vi "Query Event Log Last Entry.vi"(8 "error in (no error)":errorcluster, 11 "VISA resource name":refnum<visa-resource-name>) -> (0 "error out":errorcluster, 1 "Timestamp":string, 2 "Severity":i32, 3 "VISA resource name out":refnum<visa-resource-name>, 4 "Message":string)   [LabVIEW 2020, in "Rohde&Schwarz CMXP Base.lvlib"]
doc: "Queries the last event log.\n\nAttribute:\nRSCMXPBASE_ATTR_EVENT_LOG_LAST_ENTRIES\n\nRemote-control command:\nSENSe:ELOG:LAST?"
uses:
  <instrlib>/Rohde&Schwarz CMXP Base/Rohde&Schwarz CMXP Base.lvlib
  <instrlib>/Rohde&Schwarz CMXP Base/Private/rsidr_core.llb/rsidr_core.lvlib
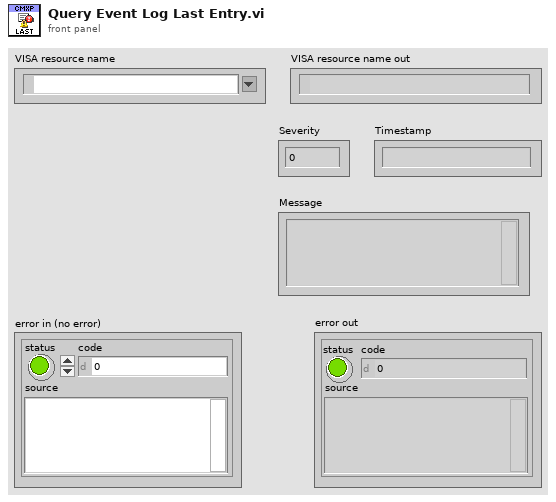
[diagram p1: front panel]
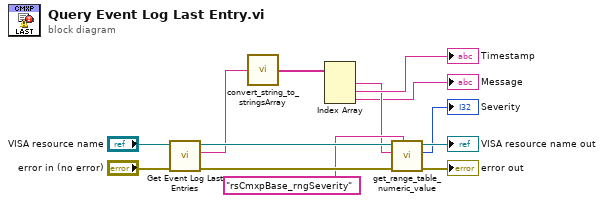
[diagram p0: block diagram]
diagram:
  n1 = call "Get Event Log Last Entries"("error in (no error)"="error in (no error)", "instrument handle"="VISA resource name") -> ("error out"=w8:errorcluster, "Event Log Last Entries"=w3:string, "instrument handle out"=w7:refnum<visa-resource-name>)  [unwired: 7 in]
  n2 = call <instrlib>:"convert_string_to_stringsArray.vi"("String in"=w3) -> ("string array out"=w5:string[])  [unwired: 3 in, 1 out]
  n3 = Index Array(array=w5) -> (element #1=w2:string, element #2=→"Timestamp":string, element #3=→"Message":string)  [unwired: 3 in]
  n4 = call <instrlib>:"get_range_table_numeric_value.vi"("Range Table ID in"="rsCmxpBase_rngSeverity", "error in"=w8, "String Value"=w2, "VISA resource name"=w7) -> ("error out"=→"error out":errorcluster, "I32 output"=→"Severity":i32, "VISA resource name out"=→"VISA resource name out":refnum<visa-resource-name>)  [unwired: 5 in]
